vi "DataBufferSizes.vi"(8 "Down Sample Ratio":u64=1 format="%_6p", 9 "Number of Samples":u64 format="%_6p", 10 "Down-Sample Mode":u32(ring) items=["RAW none"=2147483648, "None"=0, "Aggregate"=1, "Decimate"=2, "Average"=4]) -> (1 "min Buffer Size":i32 format="%_6p", 2 "Max Buffer Size":i32 format="%_6p")   [LabVIEW 2024]
doc: "This VI returns Max. and Min. Buffer sizes using Down Sampling mode and ratio value inputs.\nOutputs can then used create arrays and pass to API functions."
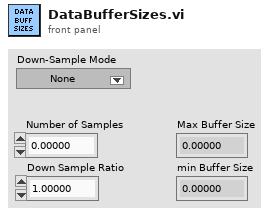
[diagram p1: front panel]
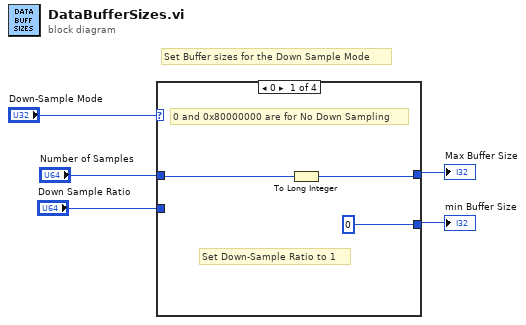
[diagram p0: block diagram]
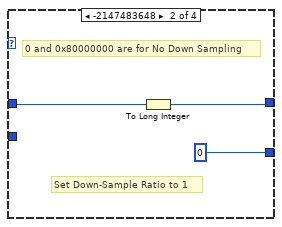
[diagram p2: hidden frame]
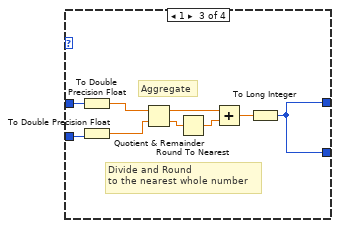
[diagram p3: hidden frame]
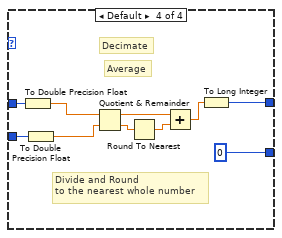
[diagram p4: hidden frame]
diagram:
  # "Set Buffer sizes for the Down Sample Mode"
  n1 = case shown="0" "Down-Sample Mode" {
    tunnel: "Down Sample Ratio" -> [_ _ w12 w21]
    tunnel: "Number of Samples" -> [w8 w11 w13 w24]
    tunnel: [w7 w10 w20 w30] -> w5
    tunnel: [0 0 w20 0] -> w4
    frame 0 {
      # "0 and 0x80000000 are for No Down Sampling"
      # "Set Down-Sample Ratio to 1"
      n2 = To Long Integer(number=w8) -> (32bit integer=w7:i32)
    }
    frame -2147483648 {
      # "0 and 0x80000000 are for No Down Sampling"
      # "Set Down-Sample Ratio to 1"
      n3 = To Long Integer(number=w11) -> (32bit integer=w10:i32)
    }
    frame 1 {
      # "Divide and Round\nto the nearest whole number"
      # "Aggregate"
      n4 = To Double Precision Float(number=w13) -> (double precision float=w16:dbl)
      n5 = To Double Precision Float(number=w12) -> (double precision float=w15:dbl)
      n6 = Quotient & Remainder(x=w16, y=w15) -> (x-y*floor(x/y)=w17:dbl, floor(x/y)=w19:dbl)
      n7 = Round To Nearest(number=w19) -> (nearest integer value=w18:dbl)
      n8 = Add(x=w17, y=w18) -> (x+y=w14:dbl)
      n9 = To Long Integer(number=w14) -> (32bit integer=w20:i32)
    }
    frame Default {
      # "Divide and Round\nto the nearest whole number"
      # "Average"
      # "Decimate"
      n10 = To Double Precision Float(number=w24) -> (double precision float=w23:dbl)
      n11 = To Double Precision Float(number=w21) -> (double precision float=w22:dbl)
      n12 = Quotient & Remainder(x=w23, y=w22) -> (x-y*floor(x/y)=w26:dbl, floor(x/y)=w28:dbl)
      n13 = Round To Nearest(number=w28) -> (nearest integer value=w27:dbl)
      n14 = Add(x=w26, y=w27) -> (x+y=w25:dbl)
      n15 = To Long Integer(number=w25) -> (32bit integer=w30:i32)
    }
  }
  "Max Buffer Size" <- w5
  "min Buffer Size" <- w4
